vi "test.vi"() -> ()   [LabVIEW 2019]
panel:
  out "Tps en nano s":u32
  out "Tick Count(Ticks) 2":u32 caption="Fin tps"
  out "D":i16
  in  "C":i16
  in  "B":i16
  in  "A":i16
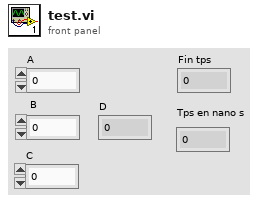
[diagram p1: front panel]
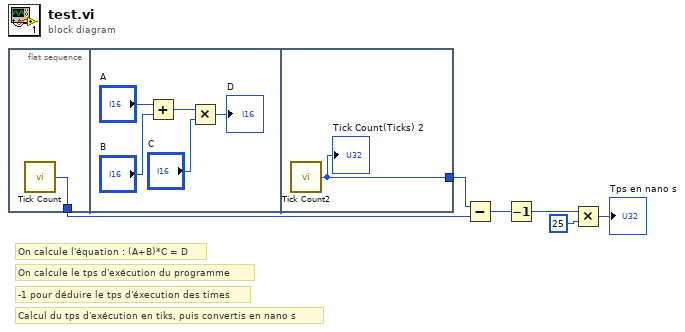
[diagram p0: block diagram]
diagram:
  # "On calcule l'équation : (A+B)*C = D"
  # "On calcule le tps d'exécution du programme"
  # "Calcul du tps d'exécution en tiks, puis convertis en nano s"
  # "-1 pour déduire le tps d'éxecution des times"
  n1 = flat-sequence {
    tunnel: [w7] -> w5
    tunnel: [w13] -> w6
    frame #0 {
      n2 = call "Tick Count"() -> ("Tick Count(Ticks)"=w7:u32)
    }
    frame #1 {
      n3 = Add(x="A", y="B") -> (x+y=w10:i16)
      n4 = Multiply(x=w10, y="C") -> (x*y=→"D":i16)
    }
    frame #2 {
      n5 = call "Tick Count2"() -> ("Tick Count(Ticks)"=w13:u32)
      "Tick Count(Ticks) 2" <- w13
    }
  }
  n6 = Subtract(x=w6, y=w5) -> (x-y=w4:u32)
  n7 = Decrement(x=w4) -> (x-1=w1:u32)
  n8 = Multiply(x=w1, y=u32 25) -> (x*y=→"Tps en nano s":u32)
